vi "Panel Routine.vi"   [LabVIEW 2018]
uses:
  <vilib>/Rock Robotics/WPI/Solenoid/WPI_SolenoidValue.ctl
  <vilib>/Rock Robotics/WPI/Solenoid/WPI_SolenoidSetEnum.vi
  Globals.vi
types:
  T1 = typedef "WPI_SolenoidValue.ctl" = enum16{"Off", "On", "Forward", "Reverse"}
  T2 = typedef "WPI_SolenoidDevRef.ctl" = cluster{"DevStatus":errorcluster, "Pneumatics Control Module":u8, "Forward Solenoid Channel":T3, "Reverse Solenoid Channel":T3}
  T3 = typedef "WPI_SolenoidChannel.ctl" = enum8{"Solenoid 0", "Solenoid 1", "Solenoid 2", "Solenoid 3", "Solenoid 4", "Solenoid 5", "Solenoid 6", "Solenoid 7", "Invalid"}
  T4 = typedef "WPI_MotorControlDeviceRef.ctl" = cluster{"DeviceStatus":errorcluster, "Type":T5, "PWM":cluster{"PWM Channel":T6, "DeadBand":T7}, "CAN":cluster{"Device Number":u8, "SetOutput VI Ref":variant, "GetOutput VI Ref":variant, "Enable VI Ref":variant, "Disable VI Ref":variant, "Data":variant}, "Invert":bool, "DIO PWM":cluster{"PWM \"Enable\" Channel":T6, "DIOChannel":T8, "PWM Rate":dbl}}
  T5 = typedef "WPI_MotorControlType.ctl" = enum16{"PWM", "CAN", "DIO PWM"}
  T6 = typedef "FPGA_DIOPWMChannel.ctl" = enum8{"PWM 0", "PWM 1", "PWM 2", "PWM 3", "PWM 4", "PWM 5", "PWM 6", "PWM 7", "PWM 8", "PWM 9", "PWM MXP 0", "PWM MXP 1", "PWM MXP 2", "PWM MXP 3", "PWM MXP 4", "PWM MXP 5", "PWM MXP 6", "PWM MXP 7", "PWM MXP 8", "PWM MXP 9", "Invalid"}
  T7 = typedef "WPI_PWMDeadband.ctl" = cluster{"Name":string, "maxPositivePwm":i32, "minPositivePwm":i32, "centerPwm":i32, "maxNegativePwm":i32, "minNegativePwm":i32, "angularRange":u16}
  T8 = typedef "FPGA_DIOChannel.ctl" = enum8{"DIO 0", "DIO 1", "DIO 2", "DIO 3", "DIO 4", "DIO 5", "DIO 6", "DIO 7", "DIO 8", "DIO 9", "DIO MXP 0", "DIO MXP 1", "DIO MXP 2", "DIO MXP 3", "DIO MXP 4", "DIO MXP 5", "DIO MXP 6", "DIO MXP 7", "DIO MXP 8", "DIO MXP 9", "DIO MXP 10", "DIO MXP 11", "DIO MXP 12", "DIO MXP 13", "DIO MXP 14", "DIO MXP 15", "SPI Port CS1", "SPI Port CS2", "SPI Port CS3", "SPI Port MISO", "SPI Port MOSI", "Invalid"}
  T9 = typedef "WPI_DigitalInputDevRef.ctl" = cluster{"DevStatus":errorcluster, "DIO Channel":T8}
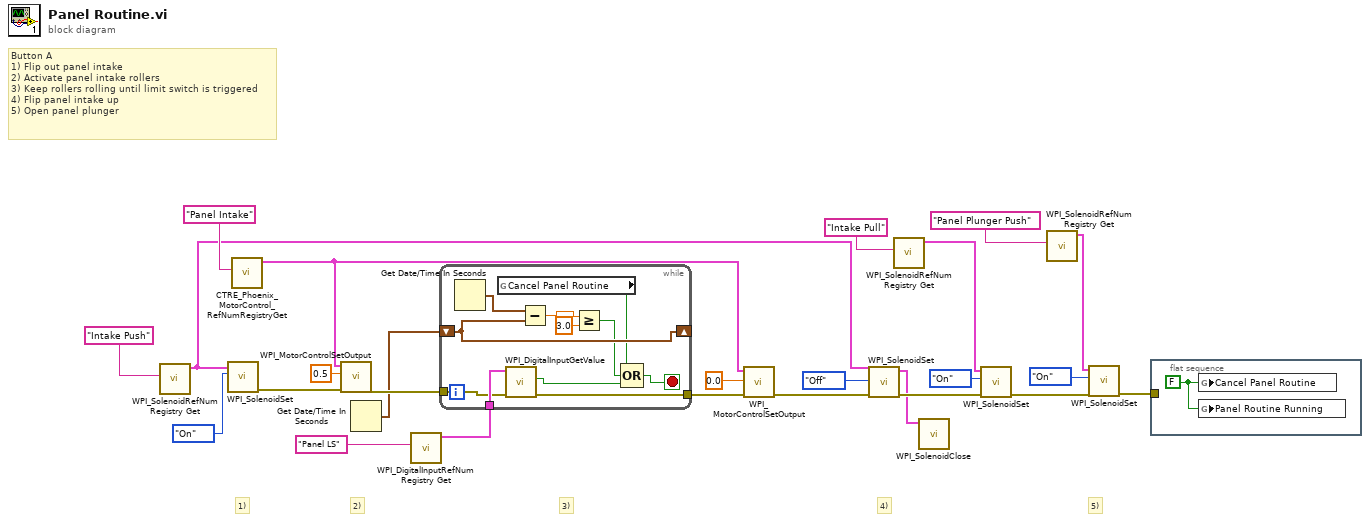
[diagram p0: block diagram]
diagram:
  # "5)"
  # "4)"
  # "3)"
  # "2)"
  # "1)"
  # "Button A\n1) Flip out panel intake\n2) Activate panel intake rollers\n3) Keep rollers rolling until limit switch is triggered\n4) Flip panel intake up\n5) Open panel plunger"
  n1 = call <vilib>:"WPI_SolenoidRefNum Registry Get.vi"("refnum name"="Intake Push") -> ("SolenoidDevRef"=w10:T2)  [unwired: 9 in, 1 out]
  n2 = call-poly <vilib>:"WPI_SolenoidSet.vi"("Value"=WPI_SolenoidValue."On", "SolenoidDevRef"=w10) -> ("error out"=w21:errorcluster)  [unwired: 1 in, 8 out]
  n3 = call <vilib>:"CTRE_Phoenix_MotorControl_RefNumRegistryGet.vi"("refnum name"="Panel Intake") -> ("PhoenixMotorControlDevRef"=w15:T4)  [unwired: 9 in, 1 out]
  n4 = call <vilib>:"WPI_MotorControlSetOutput.vi"("error in (no error)"=w21, "Output"=0.5, "MotorControlDevRef"=w15) -> ("error out"=w19:errorcluster)  [unwired: 6 in, 2 out]
  n5 = Get Date/Time In Seconds() -> (seconds since 1Jan1904=w3:timestamp)
  n6 = call <vilib>:"WPI_DigitalInputRefNum Registry Get.vi"("refnum name"="Panel LS") -> ("DigitalInputDevRef"=w23:T9)  [unwired: 9 in, 1 out]
  n7 = while {
    tunnel: w23 -> [w36]
    tunnel: w19 -> [w35]
    tunnel: [w34] -> w18
    shift-right: [w30] -> _
    shift-left: w3 -> [w30]
    stop <- w26 stop-if-true
    n8 = Get Date/Time In Seconds() -> (seconds since 1Jan1904=w33:timestamp)
    n9 = global read "Globals.vi" "Cancel Panel Routine"() -> (w28:bool)
    n10 = call <vilib>:"WPI_DigitalInputGetValue.vi"("error in (no error)"=w35, "DigitalInputDevRef"=w36) -> ("error out"=w34:errorcluster, "Value"=w27:bool)  [unwired: 7 in, 1 out]
    n11 = Subtract(x=w33, y=w30) -> (x-y=w32:dbl)
    n12 = Greater Or Equal?(x=w32, y=3.0) -> (x >= y?=w29:bool)
    n13 = Compound Arithmetic op=OR(w28, w29, w27) -> (w26:bool)
  }
  n14 = call <vilib>:"WPI_MotorControlSetOutput.vi"("error in (no error)"=w18, "Output"=0.0, "MotorControlDevRef"=w15) -> ("error out"=w16:errorcluster)  [unwired: 6 in, 2 out]
  n15 = call-poly <vilib>:"WPI_SolenoidSet.vi"("error in (no error)"=w16, "Value"=WPI_SolenoidValue."Off", "SolenoidDevRef"=w10) -> ("error out"=w13:errorcluster, "SolenoidDevRef"=w12:T2)  [unwired: 7 out]
  n16 = call <vilib>:"WPI_SolenoidRefNum Registry Get.vi"("refnum name"="Intake Pull") -> ("SolenoidDevRef"=w8:T2)  [unwired: 9 in, 1 out]
  n17 = call <vilib>:"WPI_SolenoidClose.vi"("SolenoidDevRef"=w12) -> ()  [unwired: 10 in, 1 out]
  n18 = call-poly <vilib>:"WPI_SolenoidSet.vi"("error in (no error)"=w13, "Value"=WPI_SolenoidValue."On", "SolenoidDevRef"=w8) -> ("error out"=w4:errorcluster)  [unwired: 8 out]
  n19 = call <vilib>:"WPI_SolenoidRefNum Registry Get.vi"("refnum name"="Panel Plunger Push") -> ("SolenoidDevRef"=w6:T2)  [unwired: 9 in, 1 out]
  n20 = call-poly <vilib>:"WPI_SolenoidSet.vi"("error in (no error)"=w4, "Value"=WPI_SolenoidValue."On", "SolenoidDevRef"=w6) -> ("error out"=w2:errorcluster)  [unwired: 8 out]
  n21 = flat-sequence {
    tunnel: w2 -> [_]
    frame #0 {
      w37 = FALSE ("Button X")
      n22 = global write "Globals.vi" "Cancel Panel Routine"(w37) -> ()
      n23 = global write "Globals.vi" "Panel Routine Running"(w37) -> ()
    }
  }
